vi "NanotecSMCPD.set referencing bit.vi"(0 "i ref in":refnum<vi>, 1 "axis":i32, 2 "isReferencing?":bool, 3 "ms timeout (10000)":i32=10000, 5 "error in (no error)":errorcluster) -> (14 "i ref out":refnum<vi>, 17 "timed out":bool, 19 "error out":errorcluster)   [LabVIEW 2014, in "NanotecSMCPD.lvlib"]
doc: "Sets the referencing bit (bit indicating an ongoing reference move) of an axis."
uses:
  NanotecSMCPD.lvlib
  CSCore/CSSystem/CoreDefs/CoreDefs.error_type.ctl
  CSCore/CSSystem/CoreDefs/CoreDefs.error_severity.ctl
  CSCore/CSApplicationBaseClasses/MotorBase/MotorBase.lvlib
  CSlibraries/UtilityLib/UtilityLib.lvlib
  CSCore/CSSystem/CoreLib/CoreLib.lvlib
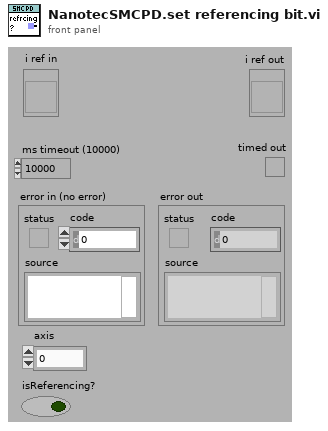
[diagram p1: front panel]
types:
  T1 = typedef "CoreDefs.error_severity.ctl" = enum16{"undefined", "information", "warning", "error", "fatal"}
  T2 = typedef "CoreDefs.error_type.ctl" = enum16{"no error", "can't load process", "can't unload process", "process does not exist", "can't install process", "can't remove process", "unknown function", "time out", "can't execute function", "duplicate queue name", "super not found", "caller queue invalid", "can't ping process", "unknown error", "VISA Error", "VISA timeout", "GPIB timeout", "GPIB error", "communication error", "data type mismatch", "can't read data from OPC server", "can't write data to OPC server", "OET error", "function not implemented", "process already exists", "invalid Shared Variable name", "error writing Shared Variable", "error reading Shared Variable", "invalid client name", "corrupt database", "unknown class", "call not authorized", "parameter out of range", "OET timeout: can't get data to modify", "invalid queue name", "requested operation incompatible with current state", "event undefined", "event disabled", "state undefined", "caller is not a friend", "EventBuilder: bad eventID", "EventBuilder: no DAQ devices", "a thread must not stop itself", "UNUSED ELEMENT4", "DiscArchiver: eventData incomplete", "DiscArchiver: eventData does not belong to run", "DiscArchiver: can't open file", "DiscArchiver: can't write to file", "DiscArchiver: available disc space low", "can't acquire semaphore", "error reading data from database", "notifier object is not existing", "can't register process", "can't unregister process", "illegal event type", "object disabled", "object already exists", "can't change state", "Instrument not found", "no connection to remote node", "invalid reference", "N/A", "UNUSED ELEMENT 1", "element not found", "illegal TCP/IP connection detected", "object does not exist", "invalid access ID", "unknown CS system", "invalid privilige", "unsupported data type", "unsupported server type", "IO server already exists", "Shared Variable already exists"}
  T3 = typedef "NanotecSMCPD.lvlib/NanotecSMCPD.i attribute.ctl" = cluster{"referencing":bool[], "stop":bool[], "AutoHalt ID":i32, "MethodQueue":refnum<queue>, "Referenced1Time?":bool[], "LastCommand ID":i32}
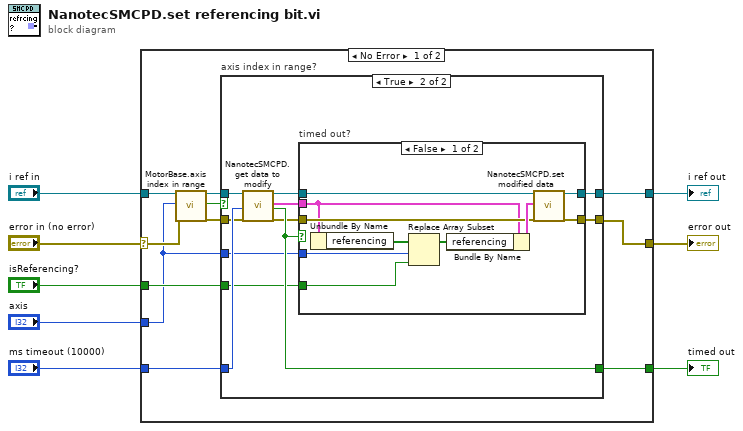
[diagram p0: block diagram]
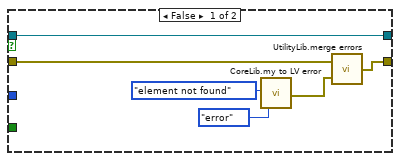
[diagram p2: hidden frame]
diagram:
  n1 = case shown="No Error" "error in (no error)" {
    selector: "error in (no error)" -> [w18 w49]
    tunnel: "ms timeout (10000)" -> [w15 _]
    tunnel: "i ref in" -> [w19 w50]
    tunnel: [w9 w49] -> w5
    tunnel: [w10 w50] -> w4
    tunnel: [w14 _] -> w3
    tunnel: "isReferencing?" -> [w13 _]
    tunnel: "axis" -> [w11 _]
    frame No Error {
      n2 = call "MotorBase.axis index in range.vi"("i ref in"=w19, "axisIndex"=w11, "error in (no error)"=w18) -> ("i ref out"=w16:refnum<vi>, "in range"=w12:bool, "error out"=w17:errorcluster)  [unwired: 14 in]
      n3 = case "axis index in range?" shown="True" w12 {
        tunnel: w16 -> [w25 w30]
        tunnel: w17 -> [w24 w31]
        tunnel: w13 -> [_ w29]
        tunnel: w15 -> [_ w36]
        tunnel: [w23 w26] -> w9
        tunnel: [_ w35] -> w14
        tunnel: w11 -> [_ w28]
        tunnel: [w25 w27] -> w10
        frame False {
          n4 = call "CoreLib.my to LV error.vi"("ErrorTypes"=CoreDefs.error_type."element not found", "severityLevel"=CoreDefs.error_severity."error") -> ("myErrorCluster"=w22:errorcluster)  [unwired: 16 in, 1 out]
          n5 = call "UtilityLib.merge errors.vi"("error2 (no error)"=w22, "error1 (no error)"=w24) -> ("error out"=w23:errorcluster)
        }
        frame True {
          n6 = call "NanotecSMCPD.get data to modify.vi"("i ref in"=w30, "ms timeout (10000)"=w36, "error in (no error)"=w31) -> ("i ref out"=w34:refnum<vi>, "i attribute"=w32:T3, "timed out"=w35:bool, "error out"=w33:errorcluster)  [unwired: 13 in]
          n7 = case "timed out?" shown="False" w35 {
            tunnel: [w46 w48] -> w27
            tunnel: w34 -> [w42 w48]
            tunnel: w33 -> [w41 w47]
            tunnel: [w45 w47] -> w26
            tunnel: w32 -> [w37 _]
            tunnel: w29 -> [w39 _]
            tunnel: w28 -> [w38 _]
            frame False {
              n8 = Unbundle By Name(w37) -> ("referencing"=w40:bool[])
              n9 = Replace Array Subset(array=w40, new element=w39, index=w38) -> (w44:bool[])
              n10 = Bundle By Name(cluster=w37, "referencing"=w44) -> (w43:T3)
              n11 = call "NanotecSMCPD.set modified data.vi"("i ref in"=w42, "i attribute"=w43, "error in (no error)"=w41) -> ("i ref out"=w46:refnum<vi>, "error out"=w45:errorcluster)  [unwired: 15 in]
            }
            frame True {
            }
          }
        }
      }
    }
    frame Error {
    }
  }
  "error out" <- w5
  "i ref out" <- w4
  "timed out" <- w3
